vi "_builtins_resize_diagram_window.vi"(8 "error in (no error)":errorcluster, 11 "VI Refnum in":refnum<vi>) -> (0 "error out":errorcluster, 3 "VI Refnum out":refnum<vi>)   [LabVIEW 2019, in "Script.lvlib"]
doc: "Resizes the block diagram window to content.\n\nCreated by: Ryan Pacini"
uses:
  Script.lvlib
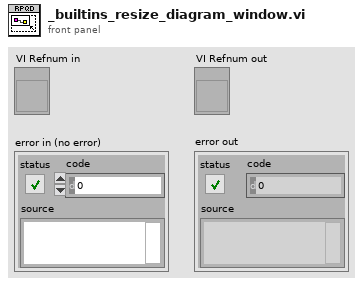
[diagram p1: front panel]
types:
  T1 = typedef "LVRectTypeDef.ctl" = cluster{"Left":i16, "Top":i16, "Right":i16, "Bottom":i16}
  T2 = typedef "LVAllMonitorsDisplayTypeDef.ctl" = cluster{"Bounds":cluster{"Left":i16, "Top":i16, "Right":i16, "Bottom":i16}, "Depth":i16}[]
  T3 = typedef "LVBoundsTypeDef.ctl" = cluster{"Width":u32, "Height":u32}
  T4 = cluster{"Left":i16, "Top":i16, "Right":i16, "Bottom":i16}
  T5 = typedef "LVPointTypeDef.ctl" = cluster{"Horizontal":i16, "Vertical":i16}
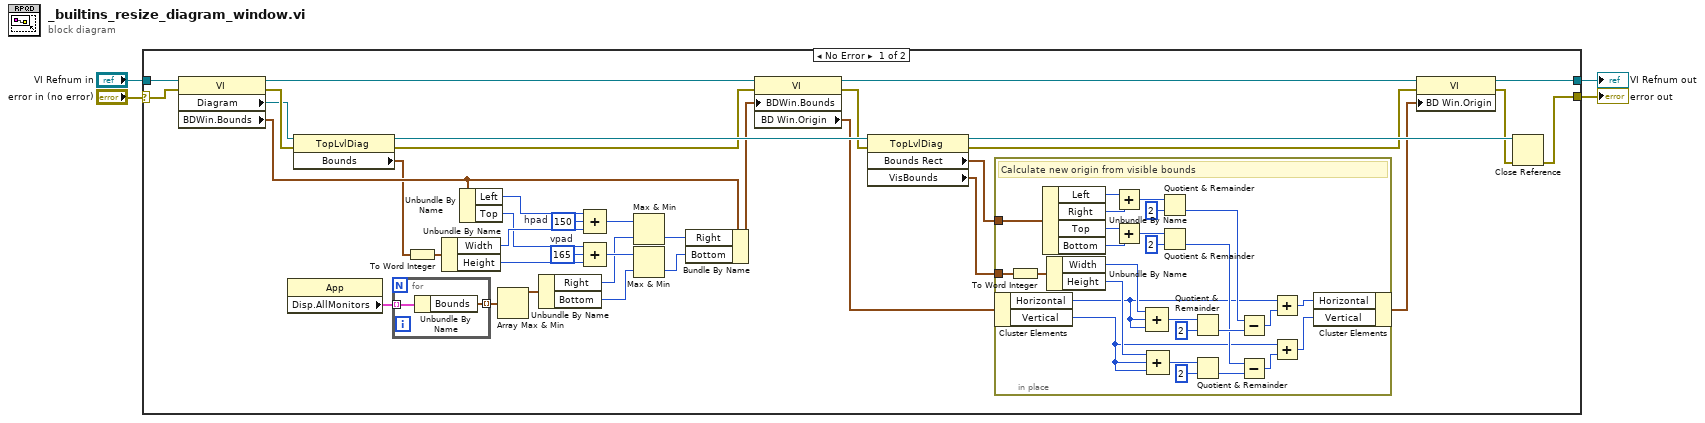
[diagram p0: block diagram]
diagram:
  n1 = case shown="No Error" "error in (no error)" {
    selector: "error in (no error)" -> [w38 w70]
    tunnel: [w40 w71] -> w4
    tunnel: "VI Refnum in" -> [w39 w71]
    tunnel: [w5 w70] -> w1
    frame No Error {
      w25 = i16 165  # vpad
      w15 = i16 150  # hpad
      n2 = property on="Property Node" class="VI"(reference=w39, error in=w38) -> (error out=w19:errorcluster, "Diagram"=w10:refnum<vi>, "BDWin.Bounds"=w34:T1)  [unwired: 1 out]
      n3 = property class="App"() -> ("Disp.AllMonitors"=w6:T2)  [unwired: 2 in, 2 out]
      n4 = property on="Property Node" class="TopLvlDiag"(reference=w10, error in=w19) -> (reference out=w36:refnum<vi>, error out=w18:errorcluster, "Bounds"=w17:T3)
      n5 = for {
        tunnel: w6 -> [w69] mode=indexing
        tunnel: [w68] -> w7 mode=indexing
        n6 = Unbundle By Name(w69) -> ("Bounds"=w68:T4)
      }
      n7 = To Word Integer(number=w17) -> (16bit integer=w28:cluster{"Width":i16, "Height":i16})
      n8 = Unbundle By Name(w28) -> ("Width"=w30:i16, "Height"=w29:i16)
      n9 = Unbundle By Name(w34) -> ("Left"=w27:i16, "Top"=w26:i16)
      n10 = Array Max & Min(array=w7) -> (max value=w24:T4)  [unwired: 3 out]
      n11 = Unbundle By Name(w24) -> ("Right"=w8:i16, "Bottom"=w9:i16)
      n12 = Compound Arithmetic op=ADD(w27, w15, w30) -> (w20:i16)
      n13 = Compound Arithmetic op=ADD(w26, w25, w29) -> (w21:i16)
      n14 = Max & Min(x=w20, y=w8) -> (min(x,y)=w22:i16)  [unwired: 1 out]
      n15 = Max & Min(x=w21, y=w9) -> (min(x,y)=w23:i16)  [unwired: 1 out]
      n16 = Bundle By Name(cluster=w34, "Right"=w22, "Bottom"=w23) -> (w16:T1)
      n17 = property on="Property Node" class="VI"(reference=w39, error in=w18, "BDWin.Bounds"=w16) -> (reference out=w35:refnum<vi>, error out=w14:errorcluster, "BD Win.Origin"=w32:T5)
      n18 = property on="Property Node" class="TopLvlDiag"(reference=w36, error in=w14) -> (reference out=w37:refnum<vi>, error out=w12:errorcluster, "Bounds Rect"=w13:T1, "VisBounds"=w31:T3)
      n19 = in-place {
        in-place-border: w13 -> [w63]
        in-place-border: w31 -> [w51]
        # "Calculate new origin from visible bounds"
        n20 = in-place-cluster #1(w32) -> ("Horizontal"=w45:i16, "Vertical"=w44:i16)
        n21 = To Word Integer(number=w51) -> (16bit integer=w50:cluster{"Width":i16, "Height":i16})
        n22 = Unbundle By Name(w63) -> ("Left"=w67:i16, "Right"=w66:i16, "Top"=w65:i16, "Bottom"=w64:i16)
        n23 = Unbundle By Name(w50) -> ("Width"=w47:i16, "Height"=w49:i16)
        n24 = Add(x=w67, y=w66) -> (x+y=w62:i16)
        n25 = Add(x=w65, y=w64) -> (x+y=w61:i16)
        n26 = Compound Arithmetic op=ADD(w47, w45, w45) -> (w46:i16)
        n27 = Compound Arithmetic op=ADD(w49, w44, w44) -> (w48:i16)
        n28 = Quotient & Remainder(x=w62, y=i16 2) -> (floor(x/y)=w57:i16)  [unwired: 1 out]
        n29 = Quotient & Remainder(x=w61, y=i16 2) -> (floor(x/y)=w54:i16)  [unwired: 1 out]
        n30 = Quotient & Remainder(x=w46, y=i16 2) -> (floor(x/y)=w58:i16)  [unwired: 1 out]
        n31 = Quotient & Remainder(x=w48, y=i16 2) -> (floor(x/y)=w56:i16)  [unwired: 1 out]
        n32 = Subtract(x=w57, y=w58) -> (x-y=w53:i16)
        n33 = Subtract(x=w54, y=w56) -> (x-y=w52:i16)
        n34 = Add(x=w45, y=w53) -> (x+y=w43:i16)
        n35 = Add(x=w44, y=w52) -> (x+y=w42:i16)
        n36 = in-place-cluster #1("Horizontal"=w43, "Vertical"=w42) -> (w33:T5)
      }
      n37 = property on="Property Node" class="VI"(reference=w35, error in=w12, "BD Win.Origin"=w33) -> (reference out=w40:refnum<vi>, error out=w11:errorcluster)
      n38 = Close Reference(reference=w37, error in (no error)=w11) -> (error out=w5:errorcluster)
    }
    frame Error {
    }
  }
  "VI Refnum out" <- w4
  "error out" <- w1
